vi "Parse Method.vi"(11 "Method text":string) -> (3 "Method Cluster":T1)   [LabVIEW 2012]
uses:
  Method.ctl
panel:
  out "Title":string
  out "About":string
  out "Stock file names":string[](array[string])
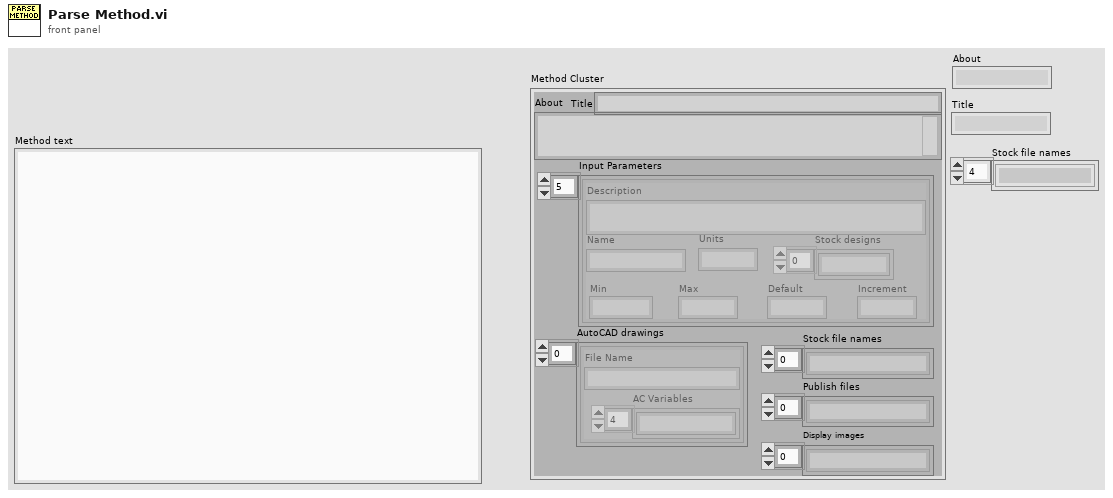
[diagram p1: front panel]
types:
  T1 = typedef "Method.ctl" = cluster{"Title":string, "About":string, "Input Parameters":cluster{"Description":string, "Name":string, "Min":string, "Max":string, "Default":string, "Units":string, "Increment":string, "Stock designs":string[]}[], "AutoCAD drawings":cluster{"File Name":string, "AC Variables":string[]}[], "Stock file names":string[], "Publish files":string[], "Display images":string[]}
  T2 = cluster{"Description":string, "Name":string, "Min":string, "Max":string, "Default":string, "Units":string, "Increment":string, "Stock designs":string[]}[]
  T3 = cluster{"File Name":string, "AC Variables":string[]}[]
  T4 = cluster{"File Name":string, "AC Variables":string[]}
  T5 = cluster{"Description":string, "Name":string, "Min":string, "Max":string, "Default":string, "Units":string, "Increment":string, "Stock designs":string[]}
  T6 = cluster{"array type (2D Dbl)[0]":string, "array type (2D Dbl)[1]":string, "array type (2D Dbl)[2]":string, "array type (2D Dbl)[3]":string, "array type (2D Dbl)[4]":string, "array type (2D Dbl)[5]":string, "array type (2D Dbl)[6]":string}
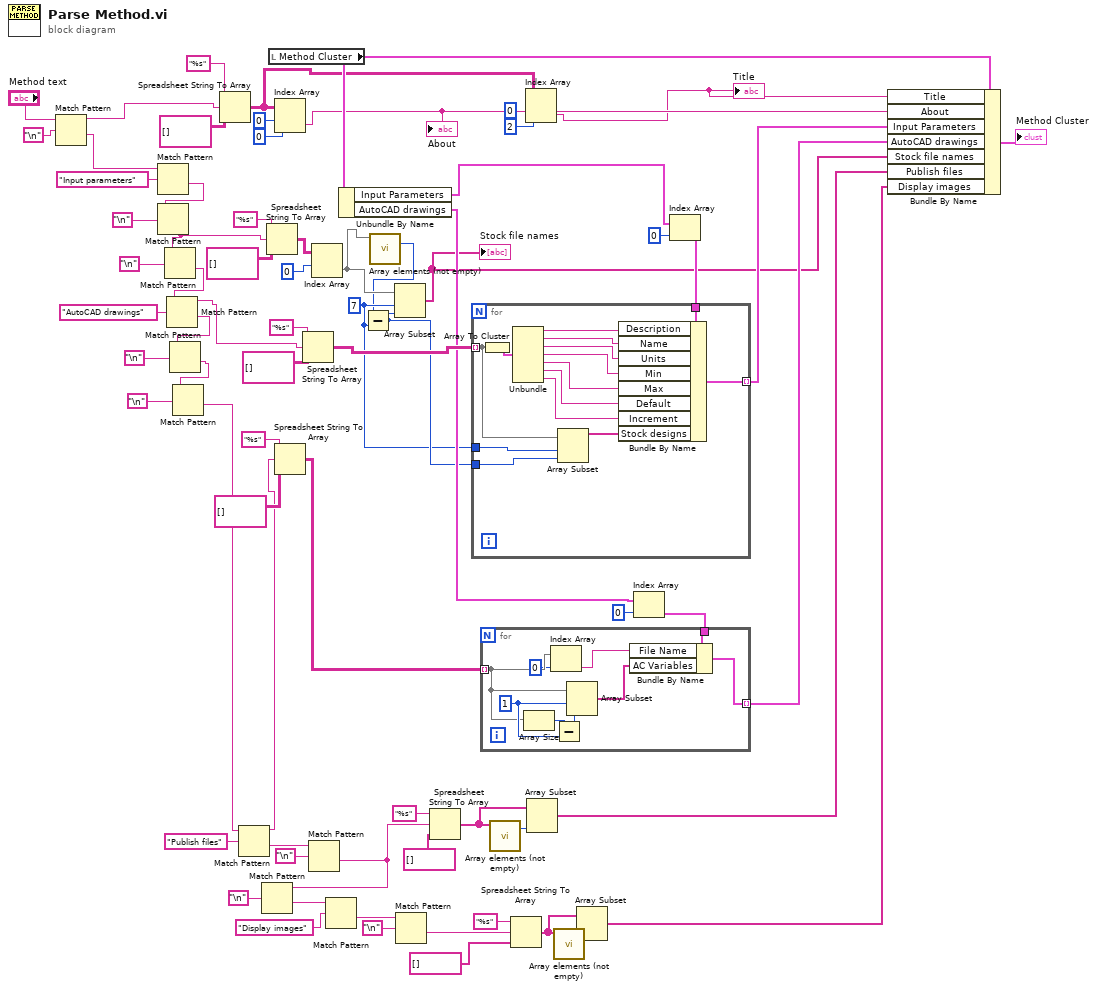
[diagram p0: block diagram]
diagram:
  w25 = 7 ("index")
  n1 = Match Pattern(string="Method text", regular expression="\n") -> (before substring=w38:string, after substring=w68:string)  [unwired: 1 in, 2 out]
  n2 = Match Pattern(string=w68, regular expression="Input parameters") -> (after substring=w46:string)  [unwired: 1 in, 3 out]
  n3 = Match Pattern(string=w46, regular expression="\n") -> (after substring=w43:string)  [unwired: 1 in, 3 out]
  n4 = Match Pattern(string=w43, regular expression="\n") -> (after substring=w63:string)  [unwired: 1 in, 3 out]
  n5 = Match Pattern(string=w63, regular expression="AutoCAD drawings") -> (before substring=w58:string, after substring=w59:string)  [unwired: 1 in, 2 out]
  n6 = Match Pattern(string=w59, regular expression="\n") -> (after substring=w62:string)  [unwired: 1 in, 3 out]
  n7 = Match Pattern(string=w62, regular expression="\n") -> (after substring=w14:string)  [unwired: 1 in, 3 out]
  n8 = Spreadsheet String To Array(format string="%s", spreadsheet string=w38, array type (2D Dbl)=string[][] []) -> (array=w30:string[][])  [unwired: 1 in]
  n9 = Match Pattern(string=w14, regular expression="Publish files") -> (before substring=w10:string, after substring=w9:string)  [unwired: 1 in, 2 out]
  n10 = Spreadsheet String To Array(format string="%s", spreadsheet string=w43, array type (2D Dbl)=string[][] []) -> (array=w42:string[][])  [unwired: 1 in]
  n11 = local read "Method Cluster"() -> (w55:T1)
  n12 = Index Array(array=w30, index (row)=0, index (col)=0 ("disabled index (col)")) -> (element=w35:string)
  "About" <- w35
  n13 = Spreadsheet String To Array(format string="%s", spreadsheet string=w10, array type (2D Dbl)=string[][] []) -> (array=w48:string[][])  [unwired: 1 in]
  n14 = Spreadsheet String To Array(format string="%s", spreadsheet string=w58, array type (2D Dbl)=string[][] []) -> (array=w53:string[][])  [unwired: 1 in]
  n15 = Match Pattern(string=w9, regular expression="\n") -> (after substring=w1:string)  [unwired: 1 in, 3 out]
  n16 = Match Pattern(string=w1, regular expression="\n") -> (after substring=w13:string)  [unwired: 1 in, 3 out]
  n17 = Index Array(array=w42, index (row)=0) -> (element=w12:string[])  [unwired: 1 in]
  n18 = Match Pattern(string=w13, regular expression="Display images") -> (after substring=w15:string)  [unwired: 1 in, 3 out]
  n19 = Unbundle By Name(w55) -> ("Input Parameters"=w31:T2, "AutoCAD drawings"=w32:T3)
  n20 = call "Array elements (not empty).vi"("1D array"=w12) -> ("# elements"=w11:i32)  [unwired: 10 in]
  n21 = Subtract(x=w11, y=w25) -> (x-y=w26:i32)
  n22 = Array Subset(array=w12, index=w25, length=w26) -> (w27:string[])
  "Stock file names" <- w27
  n23 = Match Pattern(string=w15, regular expression="\n") -> (after substring=w8:string)  [unwired: 1 in, 3 out]
  n24 = Spreadsheet String To Array(format string="%s", spreadsheet string=w1, array type (2D Dbl)=string[] []) -> (array=w6:string[])  [unwired: 1 in]
  n25 = call "Array elements (not empty).vi"("1D array"=w6) -> ("# elements"=w7:i32)  [unwired: 10 in]
  n26 = Spreadsheet String To Array(format string="%s", spreadsheet string=w8, array type (2D Dbl)=string[] []) -> (array=w4:string[])  [unwired: 1 in]
  n27 = Index Array(array=w30, index (row)=0, index (col)=2 ("disabled index (col)")) -> (element=w28:string)
  "Title" <- w28
  n28 = Array Subset(array=w6, length=w7) -> (w3:string[])  [unwired: 1 in]
  n29 = call "Array elements (not empty).vi"("1D array"=w4) -> ("# elements"=w5:i32)  [unwired: 10 in]
  n30 = Array Subset(array=w4, length=w5) -> (w2:string[])  [unwired: 1 in]
  n31 = Index Array(array=w32, index=0) -> (element=w49:T4)
  n32 = for {
    tunnel: w48 -> [w75] mode=indexing
    tunnel: [w81] -> w47 mode=indexing
    tunnel: w49 -> [w77]
    w80 = 1 ("index")
    n33 = Array Size(array=w75) -> (size(s)=w79:i32)
    n34 = Index Array(array=w75, index=0) -> (element=w73:string)
    n35 = Subtract(x=w79, y=w80) -> (x-y=w78:i32)
    n36 = Array Subset(array=w75, index=w80, length=w78) -> (w76:string[])
    n37 = Bundle By Name(cluster=w77, "File Name"=w73, "AC Variables"=w76) -> (w81:T4)
  }
  n38 = Index Array(array=w31, index=0) -> (element=w51:T5)
  n39 = for {
    tunnel: w53 -> [w85] mode=indexing
    tunnel: [w86] -> w54 mode=indexing
    tunnel: w51 -> [w84]
    tunnel: w26 -> [w83]
    tunnel: w25 -> [w82]
    n40 = Array To Cluster(array=w85) -> (cluster=w95:T6)
    n41 = Unbundle(w95) -> ("array type (2D Dbl)[0]"=w94:string, "array type (2D Dbl)[1]"=w93:string, "array type (2D Dbl)[2]"=w92:string, "array type (2D Dbl)[3]"=w91:string, "array type (2D Dbl)[4]"=w90:string, "array type (2D Dbl)[5]"=w89:string, "array type (2D Dbl)[6]"=w88:string)
    n42 = Array Subset(array=w85, index=w82, length=w83) -> (w87:string[])
    n43 = Bundle By Name(cluster=w84, "Description"=w94, "Name"=w93, "Units"=w92, "Min"=w91, "Max"=w90, "Default"=w89, "Increment"=w88, "Stock designs"=w87) -> (w86:T5)
  }
  n44 = Bundle By Name(cluster=w55, "Title"=w28, "About"=w35, "Input Parameters"=w54, "AutoCAD drawings"=w47, "Stock file names"=w27, "Publish files"=w3, "Display images"=w2) -> (→"Method Cluster":T1)
